vi "Activation Complete.vi"(8 "error in":errorcluster, 10 "Activation Complete":bool, 11 "SCADA in":refnum<class "EMS.lvclass">) -> (0 "error out":errorcluster, 3 "SCADA out":refnum<class "EMS.lvclass">)   [LabVIEW 2018, in "EMS Core.lvlib" / "EMS.lvclass"]
uses:
  EMS.lvclass
  C:/Users/Administrator/Desktop/LabVIEW EMS/EMS Generic Actor/EMS Generic/EMS Generic.lvclass
  EMS Generic Actor/EMS Generic/EMS Generic.lvclass
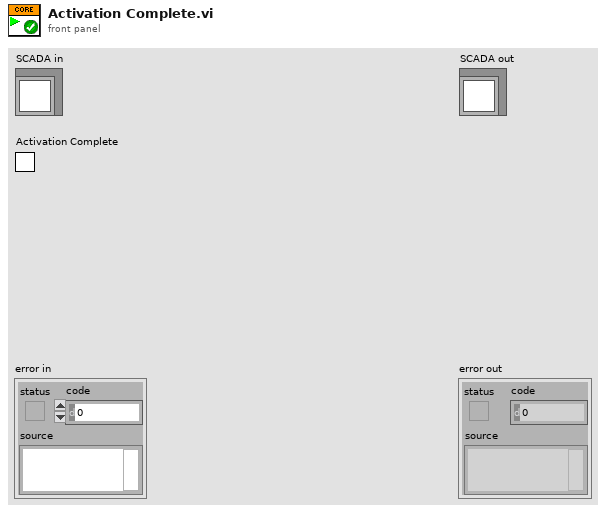
[diagram p1: front panel]
types:
  T1 = typedef "CSEISMIC DDS.lvlib/CSEISMIC DDS.lvclass/DeviceID.ctl" = string
  T2 = typedef "CSEISMIC DDS.lvlib/CSEISMIC DDS.lvclass/IED_Status.ctl" = cluster{"DeviceID":T1, "Timestamp":T3, "MicrogridID":u8, "Active":bool, "Inactive":bool, "Error":i32, "Fault":bool, "ErrorString":string}
  T3 = typedef "CSEISMIC DDS.lvlib/CSEISMIC DDS.lvclass/Timestamp.ctl" = cluster{"Seconds":u64, "Remainder":u64}
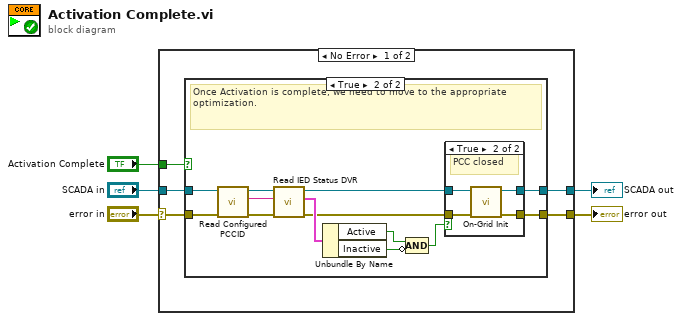
[diagram p0: block diagram]
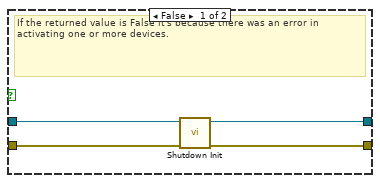
[diagram p2: hidden frame]
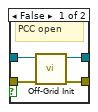
[diagram p3: hidden frame]
diagram:
  n1 = case shown="No Error" "error in" {
    selector: "error in" -> [w7 w37]
    tunnel: [w6 w37] -> w4
    tunnel: [w8 w36] -> w2
    tunnel: "SCADA in" -> [w9 w36]
    tunnel: "Activation Complete" -> [w10 _]
    frame No Error {
      n2 = case shown="True" w10 {
        tunnel: w9 -> [w14 w22]
        tunnel: [w13 w27] -> w8
        tunnel: w7 -> [w12 w20]
        tunnel: [w11 w15] -> w6
        frame False {
          # "If the returned value is False it's because there was an error in activating one or more devices."
          n3 = call "Shutdown Init.vi"("error in"=w12, "SCADA in"=w14) -> ("error out"=w11:errorcluster, "SCADA out"=w13:refnum<class "EMS.lvclass">)  [unwired: 8 in]
        }
        frame True {
          # "Once Activation is complete, we need to move to the appropriate optimization."
          n4 = call "Read Configured PCCID.vi"("error in"=w20, "EMS Generic in"=w22) -> ("error out"=w24:errorcluster, "PCCID"=w25:T1, "EMS Generic out"=w23:refnum<class "EMS.lvclass">)  [unwired: 7 in]
          n5 = call "Read IED Status DVR.vi"("error in"=w24, "DeviceID"=w25, "EMS Generic in"=w23) -> ("error out"=w19:errorcluster, "IED_Status"=w26:T2, "EMS Generic out"=w21:refnum<class "EMS.lvclass">)  [unwired: 5 in, 1 out]
          n6 = Unbundle By Name(w26) -> ("Active"=w18:bool, "Inactive"=w17:bool)
          n7 = Compound Arithmetic op=AND(w18, invert w17) -> (w16:bool)
          n8 = case shown="True" w16 {
            tunnel: [w28 w35] -> w27
            tunnel: w21 -> [w31 w33]
            tunnel: w19 -> [w30 w32]
            tunnel: [w29 w34] -> w15
            frame False {
              # "PCC open"
              n9 = call "Off-Grid Init.vi"("error in"=w30, "SCADA in"=w31) -> ("error out"=w29:errorcluster, "SCADA out"=w28:refnum<class "EMS.lvclass">)  [unwired: 8 in]
            }
            frame True {
              # "PCC closed"
              n10 = call "On-Grid Init.vi"("error in"=w32, "SCADA in"=w33) -> ("error out"=w34:errorcluster, "SCADA out"=w35:refnum<class "EMS.lvclass">)  [unwired: 8 in]
            }
          }
        }
      }
    }
    frame Error {
    }
  }
  "error out" <- w4
  "SCADA out" <- w2
